vi "Task ID.vi"(8 "error in (no error)":errorcluster, 11 "DataLogger in":refnum<class "DataLogger.lvclass">) -> (0 "error out":errorcluster, 2 "Task ID":string, 3 "DataLogger out":refnum<class "DataLogger.lvclass">)   [LabVIEW 2020, in "VolatusDataLogger.lvlib" / "DataLogger.lvclass"]
uses:
  DataLogger.lvclass
  DataLogger.lvclass/DataLogger.ctl
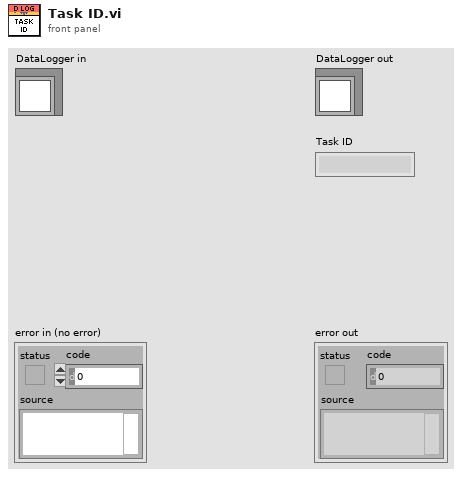
[diagram p1: front panel]
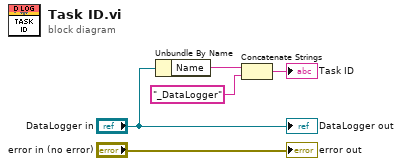
[diagram p0: block diagram]
diagram:
  n1 = Unbundle By Name("DataLogger in") -> ("Name"=w3:string)
  n2 = Concatenate Strings(w3, "_DataLogger" ("string")) -> (→"Task ID":string)
  "error out" <- "error in (no error)"
  "DataLogger out" <- "DataLogger in"
